vi "LKIF2_GetCalcDataALL.vi"(8 "error in (no error)":errorcluster {"code" format="%x"}) -> (0 "error out":errorcluster {"code" format="%x"}, 2 "OutNo":i32, 3 "CalcData":T2(array[cluster]) {"LKIF_FLOATRESULT" items=["VALID", "RANGEOVER_P", "RANGEOVER_N", "WAITING", "ALARM", "INVALID"]})   [LabVIEW 2013, in "Keyence LK-G5000.lvlib"]
uses:
  <instrlib>/Keyence LK-G5000/Keyence LK-G5000.lvlib
  <instrlib>/Keyence LK-G5000/Public/enum/LKIF_FLOATRESULT.ctl
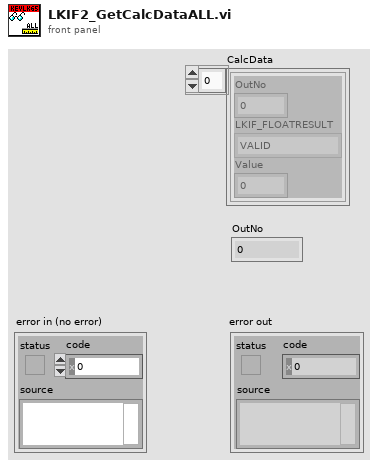
[diagram p1: front panel]
types:
  T1 = typedef "Keyence LK-G5000.lvlib/LKIF_FLOATRESULT.ctl" = i32
  T2 = cluster{"OutNo":i32, "LKIF_FLOATRESULT":T1, "Value":sgl}[]
  T3 = cluster{"OutNo":i32, "LKIF_FLOATRESULT":T1, "Value":sgl}
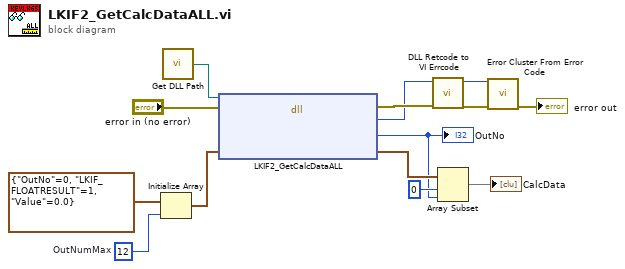
[diagram p0: block diagram]
diagram:
  w10 = 12  # OutNumMax
  n1 = Initialize Array(T3 {"OutNo"=0, "LKIF_FLOATRESULT"=1, "Value"=0.0} ("LKIF_FLOATVALUE_OUT"), w10) -> (w8:T2)
  n2 = call <instrlib>:"Get DLL Path.vi"() -> ("DLL Path"=w5:path)  [unwired: 1 in]
  n3 = dll-call lib="C:/Program Files/National Instruments/LabVIEW 2011/instr.lib/Keyence LK-G5000/LKIF2.dll" fn="LKIF2_GetCalcDataALL"(path in=w5, error in="error in (no error)", "CalcData"=w8) -> (error out=w7:errorcluster, "RC"=w6:i32, "OutNo"=w2:i32, "CalcData"=w4:T2)  [unwired: 2 in, 1 out]
  "OutNo" <- w2
  n4 = call <instrlib>:"DLL Retcode to VI Errcode.vi"("error in (no error)"=w7, "DLL Retcode"=w6) -> ("error out"=w14:errorcluster, "VI Errcode"=w13:i32)  [unwired: 8 in]
  n5 = Array Subset(array=w4, index=0 ("Žw•W"), length=w2) -> (→"CalcData":T2)
  n6 = call <vilib>:"Error Cluster From Error Code.vi"("error in (no error)"=w14, "error code (0)"=w13) -> ("error out"=→"error out":errorcluster)  [unwired: 7 in]
